vi "Local Error Handler.vi"(8 "error in (no error)":errorcluster, 11 "Boolean in":bool) -> (0 "error out":errorcluster, 3 "Boolean out":bool)   [LabVIEW 2013, in "Modbus Module editor node.lvclass"]
uses:
  Modbus Module editor node.lvclass
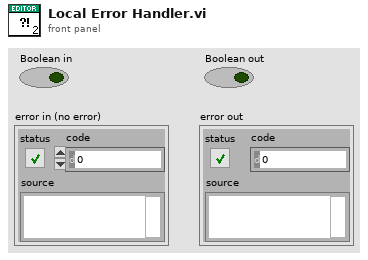
[diagram p1: front panel]
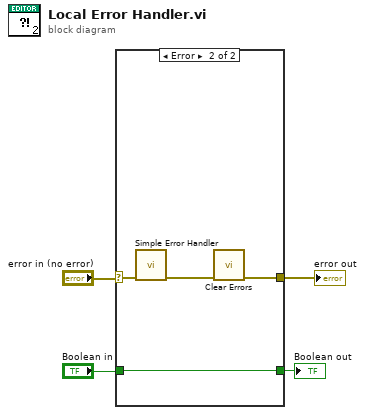
[diagram p0: block diagram]
diagram:
  n1 = case shown="Error" "error in (no error)" {
    selector: "error in (no error)" -> [w5 w9]
    tunnel: [w6 w10] -> w1
    tunnel: "Boolean in" -> [w6 w10]
    tunnel: [w5 w7] -> w2
    frame No Error {
    }
    frame Error {
      n2 = call <vilib>:"Simple Error Handler.vi"("error in (no error)"=w9) -> ("error out"=w8:errorcluster)  [unwired: 4 in, 4 out]
      n3 = call <vilib>:"Clear Errors.vi"("error in (no error)"=w8) -> ("error out"=w7:errorcluster)  [unwired: 6 in]
    }
  }
  "error out" <- w2
  "Boolean out" <- w1
